vi "Write Reading.vi"(8 "error in (no error)":errorcluster, 10 "Reading":T1={"Reading #"=0, "Readings"=[3.9289019107818604], "Reading Name"="Splice distortion", "Type"=enum."Defect", "Alarm priority"=enum."No Alarm", "Display precision"=0}, 11 "SQLite Connection in":refnum<class "Connection.lvclass">) -> (0 "error out":errorcluster, 3 "SQLite Connection":refnum<class "Connection.lvclass">)   [LabVIEW 2017, in "SQlkite Template.lvlib"]
uses:
  Beltwatch/BeltWatch 4-2-2-5/Database/SQlkite Template.lvlib
  SQ Lite Cluster Action.ctl
  Beltwatch/SourceCode/BeltWatch Reading.ctl
  Beltwatch/SourceCode/BeltWatch Event type.ctl
  Beltwatch/SourceCode/BeltWatch Alarm Priority.ctl
  <vilib>/drjdpowell/SQLite Library/SQL Connection/Connection.lvclass
  <vilib>/drjdpowell/SQLite Library/SQL Statement/SQL Statement.lvclass/SQL Statement.ctl
  <vilib>/drjdpowell/SQLite Library/SQL Connection/Connection.lvclass/Connection.ctl
  <vilib>/drjdpowell/SQLite Library/SQL Statement/Bind Integer.vi
  <vilib>/drjdpowell/SQLite Library/SQL Statement/Bind Real.vi
  <vilib>/drjdpowell/SQLite Library/SQL Statement/Error Message.vi
  <vilib>/drjdpowell/SQLite Library/SQL Statement/SQL Statement.lvclass
panel:
  out "Time 2":u32
  out "size(s)":i32
  out "Numeric":i32
  out "Valtime":u32
  out "Time":u32
  out "Array":string[](array[string])
  out "Controls[]":refnum<vi>[](array[refnum])
  out "Reading SQL":string
  out "SQLite3 type":T4(ring)
  in  "ReadingsCols":T5[](array[typedef])=[{"Include"=TRUE, "Name"="Reading #", "SQLite3 type"=enum."SQLITE_INTEGER"}, {"Include"=TRUE, "Name"="Readings", "SQLite3 type"=enum."SQLITE3_TEXT"}, {"Include"=TRUE, "Name"="Reading Name", "SQLite3 type"=enum."SQLITE3_TEXT"}, {"Include"=TRUE, "Name"="TypeVal", "SQLite3 type"=enum."SQLITE_INTEGER"}, {"Include"=TRUE, "Name"="Alarm priority", "SQLite3 type"=enum."SQLITE_INTEGER"}, {"Include"=FALSE, "Name"="Display precision", "SQLite3 type"=enum."undefined type (0)"}, {"Include"=TRUE, "Name"="TypeStr", "SQLite3 type"=enum."SQLITE3_TEXT"}, {"Include"=TRUE, "Name"="AlarmPriorityStr", "SQLite3 type"=enum."SQLITE3_TEXT"}]
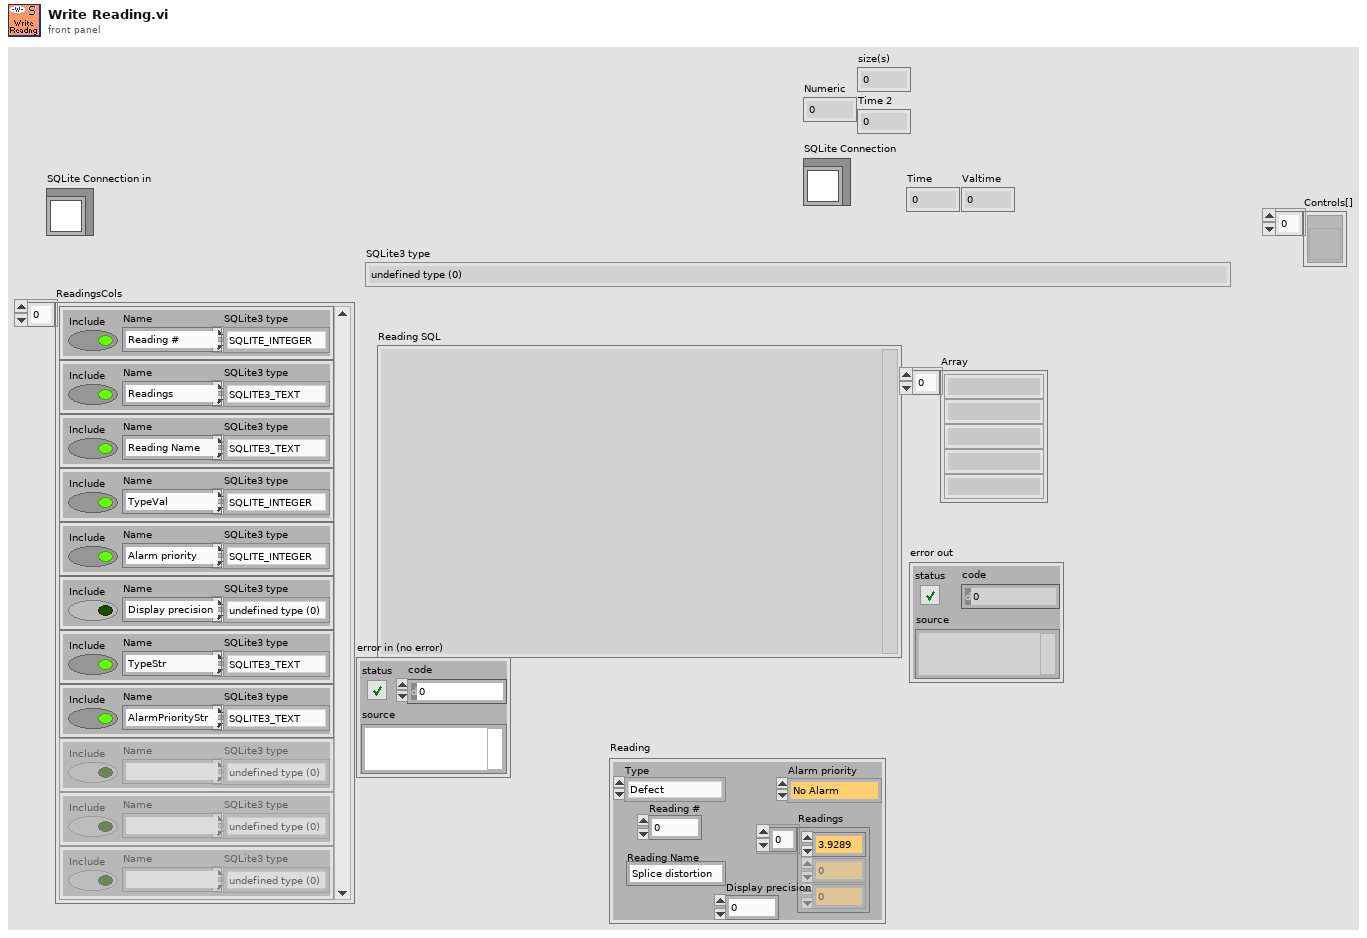
[diagram p1: front panel]
types:
  T1 = typedef "BeltWatch Reading.ctl" = cluster{"Reading #":i32, "Readings":dbl[], "Reading Name":string, "Type":T2, "Alarm priority":T3, "Display precision":i32}
  T2 = typedef "BeltWatch Event type.ctl" = enum16{"Defect", "Splice", "Break", "Rip", "Track", "Segment", "Belt", "New Splice", "Missing Splice", "None", "Free"}
  T3 = typedef "BeltWatch Alarm Priority.ctl" = enum16{"No Alarm", "High", "Medium", "Low"}
  T4 = enum32{"undefined type (0)", "SQLITE_INTEGER", "SQLITE_FLOAT", "SQLITE3_TEXT", "SQLITE_BLOB", "SQLITE_NULL", "undefined type"}
  T5 = typedef "SQlkite Template.lvlib/SQ Lite Cluster Action.ctl" = cluster{"Include":bool, "Name":string, "SQLite3 type":enum32{"undefined type (0)", "SQLITE_INTEGER", "SQLITE_FLOAT", "SQLITE3_TEXT", "SQLITE_BLOB", "SQLITE_NULL", "undefined type"}}
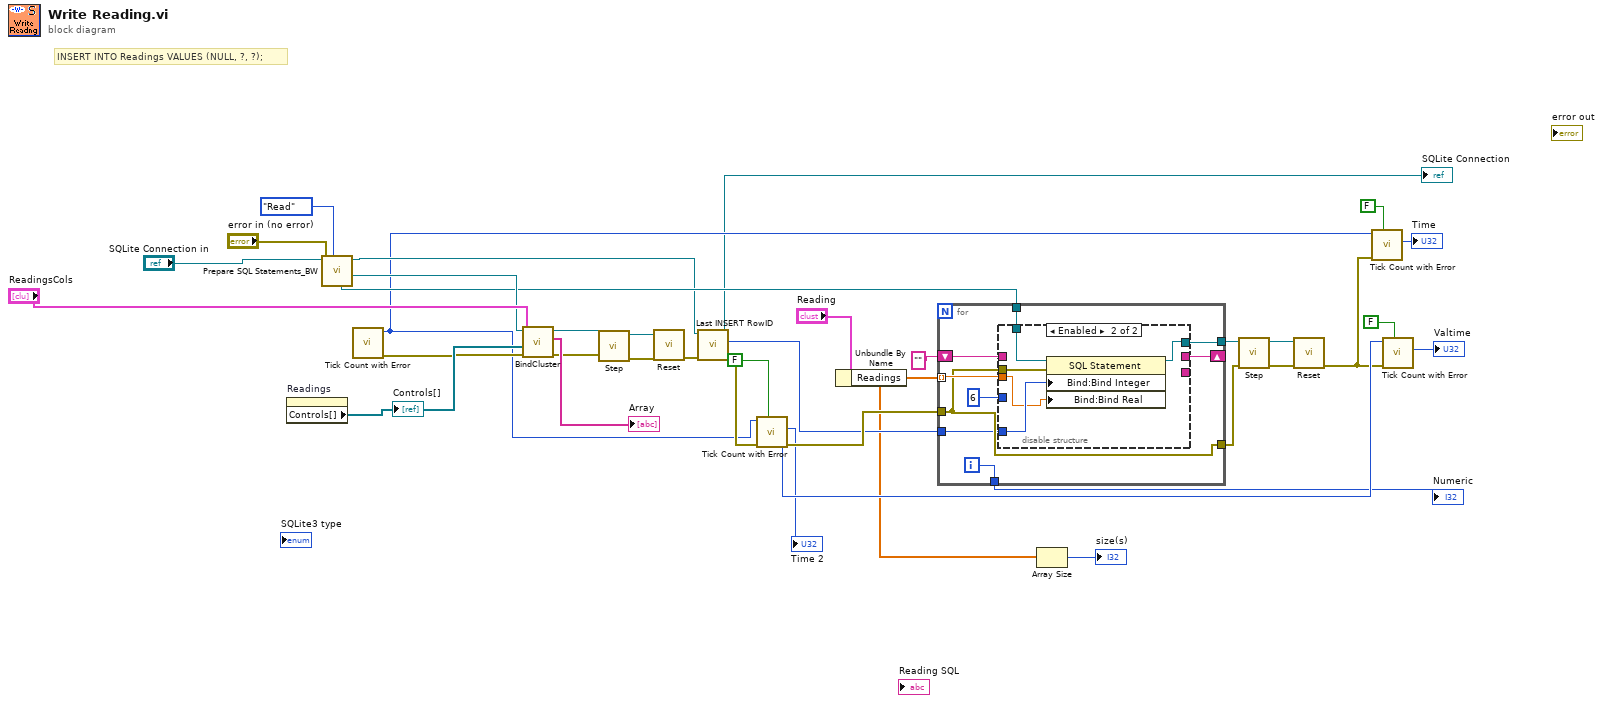
[diagram p0: block diagram]
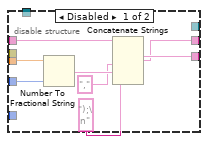
[diagram p2: hidden frame]
diagram:
  # "INSERT INTO Readings VALUES (NULL, ?, ?);"
  n1 = property on="Readings" class="Clust (strict)"() -> ("Controls[]"=w35:refnum<vi>[])  [unwired: 2 in, 2 out]
  "Controls[]" <- w35
  n2 = call "Prepare SQL Statements_BW.vi"("action"=enum16{"Init", "Read", "Finalise"}."Read", "error in (no error)"="error in (no error)", "SQLite Connection in"="SQLite Connection in") -> ("Readings"=w27:refnum<class "SQL Statement.lvclass">, "SQLite Connection out"=w10:refnum<class "Connection.lvclass">, "REadingVal"=w15:refnum<class "SQL Statement.lvclass">)  [unwired: 4 in, 2 out]
  n3 = call "Tick Count with Error.vi"() -> ("error out"=w32:errorcluster, "millisecond timer value"=w2:u32)  [unwired: 9 in, 1 out]
  n4 = call "BindCluster.vi"("error in (no error)"=w32, "Controls[]"=w35, "Cols"="ReadingsCols", "SQL Statement in"=w27) -> ("error out"=w22:errorcluster, "Array"=→"Array":string[], "SQL Statement out"=w26:refnum<class "SQL Statement.lvclass">)  [unwired: 4 in, 1 out]
  n5 = call <vilib>:"Step.vi"("error in (no error)"=w22, "SQL Statement in"=w26) -> ("error out"=w28:errorcluster, "SQL Statement"=w29:refnum<class "SQL Statement.lvclass">)  [unwired: 7 in, 1 out]
  n6 = call <vilib>:"Reset.vi"("error in (no error)"=w28, "SQL Statement in"=w29) -> ("error out"=w25:errorcluster)  [unwired: 8 in, 1 out]
  n7 = call <vilib>:"Last INSERT RowID.vi"("error in (no error)"=w25, "SQLite Connection in"=w10) -> ("error out"=w20:errorcluster, "Last INSERT RowID"=w14:i64, "SQLite Connection"=→"SQLite Connection":refnum<class "Connection.lvclass">)  [unwired: 7 in]
  n8 = call "Tick Count with Error.vi"("UsePrevious"=FALSE, "error in (no error)"=w20, "millisecond val in"=w2) -> ("error out"=w19:errorcluster, "Time"=→"Time 2":u32, "millisecond timer value"=w18:u32)  [unwired: 6 in]
  n9 = Unbundle By Name("Reading") -> ("Readings"=w8:dbl[])
  n10 = for {
    tunnel: w8 -> [w46] mode=indexing
    shift-right: [w44] -> _
    shift-left: "" -> [w43]
    tunnel: w19 -> [w42]
    tunnel: [w42] -> w5
    tunnel: w15 -> [w41]
    tunnel: w14 -> [w40]
    tunnel: [w39] -> w12
    tunnel: [w38] -> w9
    i -> [w38]
    n11 = disable-structure shown="Enabled" {
      disable-tunnel: w46 -> [w54 w56]
      disable-tunnel: i16 6 ("precision (6)") -> [w53 _]
      disable-tunnel: _ -> [w52 _]
      disable-tunnel: [w48 _] -> w44
      disable-tunnel: w43 -> [w47 _]
      disable-tunnel: w42 -> [_ w59]
      disable-tunnel: w41 -> [_ w58]
      disable-tunnel: w40 -> [_ w57]
      disable-tunnel: [_ w55] -> w39
      frame Disabled {
        n12 = Number To Fractional String(number=w54, precision (6)=w53) -> (F-format string=w51:string)  [unwired: 2 in]
        n13 = Concatenate Strings(w47, w52, "," ("string"), w51, ");\n" ("string")) -> (w48:string)  [unwired: 1 in]
      }
      frame Enabled {
        n14 = property class="SQL Statement"(reference=w58, error in=w59, "Bind:Bind Integer"=w57, "Bind:Bind Real"=w56) -> (reference out=w55:refnum<class "SQL Statement.lvclass">)  [unwired: 1 out]
      }
    }
  }
  "Numeric" <- w9
  n15 = Array Size(array=w8) -> (size(s)=→"size(s)":i32)
  n16 = call <vilib>:"Step.vi"("error in (no error)"=w5, "SQL Statement in"=w12) -> ("error out"=w13:errorcluster, "SQL Statement"=w11:refnum<class "SQL Statement.lvclass">)  [unwired: 7 in, 1 out]
  n17 = call <vilib>:"Reset.vi"("error in (no error)"=w13, "SQL Statement in"=w11) -> ("error out"=w6:errorcluster)  [unwired: 8 in, 1 out]
  n18 = call "Tick Count with Error.vi"("UsePrevious"=FALSE, "error in (no error)"=w6, "millisecond val in"=w2) -> ("Time"=→"Time":u32)  [unwired: 6 in, 2 out]
  n19 = call "Tick Count with Error.vi"("UsePrevious"=FALSE, "error in (no error)"=w6, "millisecond val in"=w18) -> ("Time"=→"Valtime":u32)  [unwired: 6 in, 2 out]
